vi "Launcher.vi"() -> ()   [LabVIEW 2019]
uses:
  UI Actor/UI Actor.lvclass
  C:/Program Files/National Instruments/LabVIEW 2019/vi.lib/ActorFramework/Actor/Actor.lvclass
  UI Actor/UI Actor.lvclass/UI Actor.ctl
  UI Actor/Write Coins.vi
  UI Actor/Write Msj.vi
  UI Actor/Write Products.vi
  <vilib>/ActorFramework/Actor/Actor.lvclass
panel:
  in  "Products":enum16{"Coca", "Nestle"}(ring)
  in  "Msj":enum16{"ESP", "ING"}(ring)
  in  "Coins":enum16{"MXN", "USD"}(ring)
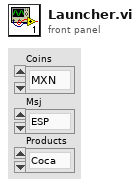
[diagram p1: front panel]
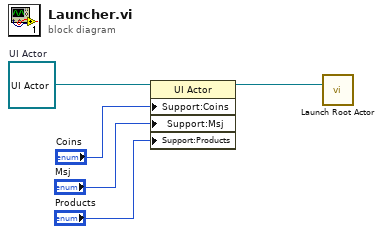
[diagram p0: block diagram]
diagram:
  w5 = refnum<class "UI Actor.lvclass"> refnum  # UI Actor
  n1 = property class="UI Actor"(reference=w5, "Support:Coins"="Coins", "Support:Msj"="Msj", "Support:Products"="Products") -> (reference out=w4:refnum<class "UI Actor.lvclass">)  [unwired: 1 in, 1 out]
  n2 = call <vilib>:"Launch Root Actor.vi"("Actor"=w4) -> ()  [unwired: 9 in, 2 out]
